vi "HEWH RLT PRAT.vi"() -> ()   [LabVIEW 2023] (continued)
            n517 = call <vilib>:"Add State(s) to Queue__jki_lib_state_machine.vi"("State(s) in (\"\")"=w1428) -> ("States Out"=w1427:string)  [unwired: 14 in]
          }
          frame "Data: Update Data Path C" {
            n518 = Unbundle By Name(w1451) -> ("Display Data (RLT).Station Label Display"=w1450:string)
            n519 = case shown="True" "New File Per CycC" {
              tunnel: w1456 -> [w1461 w1479]
              tunnel: w1455 -> [w1462 w1471]
              tunnel: [w1462 w1470] -> w1454
              tunnel: [w1460 w1467] -> w1453
              tunnel: w1450 -> [_ w1465]
              frame False {
                n520 = Bundle By Name(cluster=w1461, "File Locations C.New Summary Created"=FALSE) -> (w1460:T88)
              }
              frame True {
                # "I re-purposed this control. It now\ntriggers a header write in \"Data:\nSave\""
                # "I couldnt use a local to pass data due to UI Button"
                n521 = local read "Appliance Details C"() -> (w1464:T5)
                n522 = property on="Cycle Count Display" class="DigNum (strict)"() -> ("Value"=w1466:i32)  [unwired: 2 in, 2 out]
                n523 = Unbundle By Name(w1479) -> ("Core HEWH Data Input C.LV Program"=w1463:T25, "File Locations C"=w1474:T3)
                n524 = Unbundle By Name(w1464) -> ("Appliance Common.TR Number:"=w1477:string, "Appliance Common.Lab ID:"=w1476:string, "Appliance Common.Serial Number:"=w1475:string)
                n525 = Bundle By Name(cluster=T31 {"Appliance Details"={"FileVersionInfo"={"FileVersion"="", "ProductName"="", "InternalName"="", "CompanyName"="", "LegalCopyright"="", "FileDescription"=""}, "Dishwasher Info"={"Open Cup Weight (gm):"=0.0, "Auto Cup Weight (gm):"=0.0, "Detergent-Dish:"="", "Inlet Temperature-Dish:"="", "Cycle Mode-Dish:"="", "Unit Control-Dish:"="", "Manufacturer-Dish:"=""}, "Washer Info"={"Hot Water Temperature (Fahrenheit):"="", "Cold Water Temperature (Fahrenheit):"="", "Capacity (cu.ft):"=0.0, "Initial Cloth Weight:"=0.0, "Cloth Lot:"=0, "Model Family:"="", "Program Name:"="", "Cycle Selection:"="", "Wash Temperature:"="", "Rinse Temperature:"="", "Load Size:"=""}, "File Name Output Array"=[], "Calibration Output Array"=[], "Appliance Common"={"Engineer:"="", "Model Number:"="", "Serial Number:"="", "Comments:"="", "Station ID:"="", "Technician:"="", "TR Number:"="", "Lab ID:"="", "Voltage:"="", "Water Pressure (PSI):"="", "Test Date:"="", "Computer Name:"="", "IP Address:"="", "Ambient RH:"="", "Frequency:"="", "Build:"="", "Filename:"="", "Test Type:"="", "Load Run #:"=0, "Ambient Temperature (F):"="", "File Path:"=path "", "Cycles Per Year"=60}, "Water Heater"={"Heating Mode:"=""}, "Dryer"={"Heat Setting:"="", "Washer Water Temperature (60 ± 5°F):"=60, "Water Hardness (PPM):"=17, "Dryness Setting:"="", "Dryer Type:"="", "Exhaust:"="", "Drying Cycle:"="", "Load Type:"="", "Nominal Load Weight"="", "Dryer Initial IMC Data"={"Measured IMC (lbs)"=7.0, "Actual Initial RMC (%)"=7.0, "RMC (Desired %)"=100.0, "Bone Dry Wt(lbs)"=7.0, "Tolerance(%)"=5.0, "Actual Final RMC (%)"=0.0, "CEF (lbf/kWh)"=0.0, "Minimum Weight (lbf)"=0.0, "Average Weight (lbf)"=0.0, "Maximum Weight (lbf)"=0.0, "Measured IMC In Range?"=FALSE, "Moisture Reduction Factor"=55.5, "Field Use Factor"=1.04, "Empty Dryer Cold Weigth"=0.0, "Energy Standard"=enum."D2-Automatic Dryer", "Weight Cloth (lbs)"=0.0, "Relative Moisture Content (%)"=0.0, "Relative Moisture Content - Avg (%)"=0.0}}}, "Display Data (RLT)"={"Status Color"=0, "Serial Number Display"="", "Cycle Count Display"=0, "Station Label Display"="", "Current Run Start Time Display"=0.0, "Board ID Display"="", "RPM Display"=0, "Current Display"=0.0, "Current Path Display"=path "", "Saving Display"=FALSE, "Unit Type Display"=enum."", "Total Time On Display"=0.0, "UI Button"=FALSE}} ("Initialize.Washer In"), "Appliance Details.Appliance Common.TR Number:"=w1477, "Appliance Details.Appliance Common.Lab ID:"=w1476, "Appliance Details.Appliance Common.Serial Number:"=w1475, "Display Data (RLT).Station Label Display"=w1465, "Display Data (RLT).Cycle Count Display"=w1466) -> (w1473:T31)
                n526 = call "Save File Format All Folders.vi"("LV Program"=w1463, "error in (no error)"=w1471, "Initialize.Washer In"=w1473, "File Locations In"=w1474) -> ("error out"=w1470:errorcluster, "New File?"=w1469:bool, "File Locations Out"=w1472:T3)  [unwired: 5 in]
                n527 = Bundle By Name(cluster=w1479, "File Locations C"=w1472) -> (w1468:T88)
                n528 = Bundle By Name(cluster=w1468, "File Locations C.New Summary Created"=w1469) -> (w1467:T88)
              }
            }
            n529 = call <vilib>:"Add State(s) to Queue__jki_lib_state_machine.vi"("State(s) in (\"\")"=w1458) -> ("States Out"=w1457:string)  [unwired: 14 in]
          }
          frame "Data: Update Data Path D" {
            n530 = case shown="True" "New File Per CycD" {
              tunnel: w1485 -> [w1490 w1509]
              tunnel: w1484 -> [w1491 w1501]
              tunnel: [w1491 w1500] -> w1483
              tunnel: [w1489 w1497] -> w1482
              tunnel: w1480 -> [_ w1494]
              frame False {
                n531 = Bundle By Name(cluster=w1490, "File Locations D.New Summary Created"=FALSE) -> (w1489:T88)
              }
              frame True {
                # "I re-purposed this control. It now\ntriggers a header write in \"Data:\nSave\""
                # "I couldnt use a local to pass data due to UI Button"
                n532 = local read "Appliance Details D"() -> (w1495:T5)
                n533 = Unbundle By Name(w1494) -> ("Display Data (RLT).Station Label Display"=w1493:string)
                n534 = property on="Cycle Count Display" class="DigNum (strict)"() -> ("Value"=w1496:i32)  [unwired: 2 in, 2 out]
                n535 = Unbundle By Name(w1509) -> ("Core HEWH Data Input D.LV Program"=w1492:T25, "File Locations D"=w1504:T3)
                n536 = Unbundle By Name(w1495) -> ("Appliance Common.TR Number:"=w1507:string, "Appliance Common.Lab ID:"=w1506:string, "Appliance Common.Serial Number:"=w1505:string)
                n537 = Bundle By Name(cluster=T31 {"Appliance Details"={"FileVersionInfo"={"FileVersion"="", "ProductName"="", "InternalName"="", "CompanyName"="", "LegalCopyright"="", "FileDescription"=""}, "Dishwasher Info"={"Open Cup Weight (gm):"=0.0, "Auto Cup Weight (gm):"=0.0, "Detergent-Dish:"="", "Inlet Temperature-Dish:"="", "Cycle Mode-Dish:"="", "Unit Control-Dish:"="", "Manufacturer-Dish:"=""}, "Washer Info"={"Hot Water Temperature (Fahrenheit):"="", "Cold Water Temperature (Fahrenheit):"="", "Capacity (cu.ft):"=0.0, "Initial Cloth Weight:"=0.0, "Cloth Lot:"=0, "Model Family:"="", "Program Name:"="", "Cycle Selection:"="", "Wash Temperature:"="", "Rinse Temperature:"="", "Load Size:"=""}, "File Name Output Array"=[], "Calibration Output Array"=[], "Appliance Common"={"Engineer:"="", "Model Number:"="", "Serial Number:"="", "Comments:"="", "Station ID:"="", "Technician:"="", "TR Number:"="", "Lab ID:"="", "Voltage:"="", "Water Pressure (PSI):"="", "Test Date:"="", "Computer Name:"="", "IP Address:"="", "Ambient RH:"="", "Frequency:"="", "Build:"="", "Filename:"="", "Test Type:"="", "Load Run #:"=0, "Ambient Temperature (F):"="", "File Path:"=path "", "Cycles Per Year"=60}, "Water Heater"={"Heating Mode:"=""}, "Dryer"={"Heat Setting:"="", "Washer Water Temperature (60 ± 5°F):"=60, "Water Hardness (PPM):"=17, "Dryness Setting:"="", "Dryer Type:"="", "Exhaust:"="", "Drying Cycle:"="", "Load Type:"="", "Nominal Load Weight"="", "Dryer Initial IMC Data"={"Measured IMC (lbs)"=7.0, "Actual Initial RMC (%)"=7.0, "RMC (Desired %)"=100.0, "Bone Dry Wt(lbs)"=7.0, "Tolerance(%)"=5.0, "Actual Final RMC (%)"=0.0, "CEF (lbf/kWh)"=0.0, "Minimum Weight (lbf)"=0.0, "Average Weight (lbf)"=0.0, "Maximum Weight (lbf)"=0.0, "Measured IMC In Range?"=FALSE, "Moisture Reduction Factor"=55.5, "Field Use Factor"=1.04, "Empty Dryer Cold Weigth"=0.0, "Energy Standard"=enum."D2-Automatic Dryer", "Weight Cloth (lbs)"=0.0, "Relative Moisture Content (%)"=0.0, "Relative Moisture Content - Avg (%)"=0.0}}}, "Display Data (RLT)"={"Status Color"=0, "Serial Number Display"="", "Cycle Count Display"=0, "Station Label Display"="", "Current Run Start Time Display"=0.0, "Board ID Display"="", "RPM Display"=0, "Current Display"=0.0, "Current Path Display"=path "", "Saving Display"=FALSE, "Unit Type Display"=enum."", "Total Time On Display"=0.0, "UI Button"=FALSE}} ("Initialize.Washer In"), "Appliance Details.Appliance Common.TR Number:"=w1507, "Appliance Details.Appliance Common.Lab ID:"=w1506, "Appliance Details.Appliance Common.Serial Number:"=w1505, "Display Data (RLT).Station Label Display"=w1493, "Display Data (RLT).Cycle Count Display"=w1496) -> (w1503:T31)
                n538 = call "Save File Format All Folders.vi"("LV Program"=w1492, "error in (no error)"=w1501, "Initialize.Washer In"=w1503, "File Locations In"=w1504) -> ("error out"=w1500:errorcluster, "New File?"=w1499:bool, "File Locations Out"=w1502:T3)  [unwired: 5 in]
                n539 = Bundle By Name(cluster=w1509, "File Locations D"=w1502) -> (w1498:T88)
                n540 = Bundle By Name(cluster=w1498, "File Locations D.New Summary Created"=w1499) -> (w1497:T88)
              }
            }
            n541 = call <vilib>:"Add State(s) to Queue__jki_lib_state_machine.vi"("State(s) in (\"\")"=w1487) -> ("States Out"=w1486:string)  [unwired: 14 in]
          }
          frame "Data: Update RLT Channels" {
            # "Update the RLT Station Channels Control"
            n542 = Unbundle By Name(w1538) -> ("Core HEWH Data Input A.LV Program"=w1534:T25, "A Data Array"=w1518:string[][], "B Data Array"=w1517:string[][], "C Data Array"=w1516:string[][], "D Data Array"=w1515:string[][], "File Locations A"=w1537:T3, "File Locations B"=w1536:T3, "File Locations C"=w1510:T3, "File Locations D"=w1535:T3, "Core HEWH Data Input D"=w1523:T13, "Core HEWH Data Input C"=w1525:T13, "Core HEWH Data Input B"=w1526:T13, "Core HEWH Data Input A"=w1527:T13)
            "Station A" <- w1518
            "Station B" <- w1517
            "Station C" <- w1516
            "Station D" <- w1515
            "Station A SO Display" <- w1518
            "Station B SO Display" <- w1517
            "Station C SO Display" <- w1516
            "Station D SO Display" <- w1515
            n543 = local read "Condition B"() -> (w1513:T2)
            n544 = local read "Condition A"() -> (w1514:T2)
            n545 = local read "Station D Test Sequence"() -> (w1519:T15[])
            n546 = local read "Station A Test Sequence"() -> (w1522:T15[])
            n547 = local read "Station B Test Sequence"() -> (w1521:T15[])
            n548 = local read "Current Draw Parameters"() -> (w1532:T48)
            n549 = local read "Station C Test Sequence"() -> (w1520:T15[])
            n550 = call <vilib>:"Add State(s) to Queue__jki_lib_state_machine.vi"("State(s) in (\"\")"=w1540) -> ("States Out"=w1539:string)  [unwired: 14 in]
            n551 = local read "Condition C"() -> (w1512:T2)
            n552 = local read "Condition D"() -> (w1511:T2)
            n553 = local write "File Locations A"(w1537) -> ()
            n554 = local write "File Locations B"(w1536) -> ()
            n555 = local write "File Locations C"(w1510) -> ()
            n556 = local write "File Locations D"(w1535) -> ()
            n557 = call "HEWH Update Draw Sequence Data.vi"("Core HEWH Data Input A"=w1527, "Station A Test Sequence"=w1522, "Condition B"=w1513, "Station B Test Sequence"=w1521, "Draw Parameters"=w1532, "error in (no error)"=w1533, "Core HEWH Data Input B"=w1526, "Station C Test Sequence"=w1520, "Condition A"=w1514, "Condition C"=w1512, "Core HEWH Data Input C"=w1525, "Station D Test Sequence"=w1519, "Core HEWH Data Input D"=w1523, "Condition D"=w1511) -> ("Core HEWH Data Output"=w1528:T13, "Core HEWH Data Output 2"=w1529:T13, "Core HEWH Data Output 3"=w1530:T13, "Core HEWH Data Output 4"=w1531:T13, "error out"=w1524:errorcluster)  [unwired: 1 in]
            n558 = case shown="\"HEWH RLT\"" w1534 {
              tunnel: w1518 -> [_ w1552]
              tunnel: w1517 -> [_ w1549]
              tunnel: w1516 -> [_ w1548]
              tunnel: w1515 -> [_ w1547]
              frame Default {
              }
              frame "HEWH RLT" {
                n559 = local read "DAQ for B"() -> (w1546:bool)
                n560 = local read "DAQ for D"() -> (w1544:bool)
                n561 = local read "DAQ for A"() -> (w1551:bool)
                n562 = local read "DAQ for C"() -> (w1545:bool)
                n563 = call "HEWH RLT Get Current.vi"("DAQ for A"=w1551, "A Data Array"=w1552) -> ("Current"=w1550:dbl)  [unwired: 8 in, 1 out]
                n564 = call "HEWH RLT Get Current.vi"("DAQ for A"=w1546, "A Data Array"=w1549) -> ("Current"=w1543:dbl)  [unwired: 8 in, 1 out]
                n565 = call "HEWH RLT Get Current.vi"("DAQ for A"=w1545, "A Data Array"=w1548) -> ("Current"=w1542:dbl)  [unwired: 8 in, 1 out]
                n566 = call "HEWH RLT Get Current.vi"("DAQ for A"=w1544, "A Data Array"=w1547) -> ("Current"=w1541:dbl)  [unwired: 8 in, 1 out]
                n567 = local write "Current (D)"(w1541) -> ()
                n568 = local write "Current (A)"(w1550) -> ()
                n569 = local write "Current (B)"(w1543) -> ()
                n570 = local write "Current (C)"(w1542) -> ()
              }
            }
            n571 = local write "Core HEWH Data Input B"(w1529) -> ()
            n572 = local write "Core HEWH Data Input A"(w1528) -> ()
            n573 = local write "Core HEWH Data Input C"(w1530) -> ()
            n574 = local write "Core HEWH Data Input D"(w1531) -> ()
          }
          frame "Show Data A" {
            n575 = Unbundle By Name(w1568) -> ("Plot Array A"=w1571:dbl[][], "A Data Array"=w1561:string[][], "File Locations A.New Summary Created"=w1562:bool, "Core HEWH Data Input A.LV Program"=w1554:T25)
            n576 = call <vilib>:"Add State(s) to Queue__jki_lib_state_machine.vi"("State(s) in (\"\")"=w1573) -> ("States Out"=w1572:string)  [unwired: 14 in]
            n577 = Transpose 2D Array(2D array=w1561) -> (transposed array=w1560:string[][])
            n578 = case shown="Default" w1554 {
              tunnel: [TRUE ("Reset After 24hrs") FALSE ("Reset After 24hrs")] -> w1555
              frame Default {
              }
              frame "PRAT", "HEWH RLT" {
              }
            }
            n579 = call "UTILITY Create Plot Array.vi"("Save Data"=w1560, "Plot Array in"=w1571) -> ("Plot Array out"=w1559:dbl[][])  [unwired: 8 in, 1 out]
            n580 = call "UTILITY MultiPlot.vi"("Y-Axis-2"="Y-Axis2 - Station A", "Y-Axis-1"="Y-Axis1 - Station A", "X-Axis"="X-Axis - Station A", "Save Data"=w1560, "Plot Array"=w1571) -> ("Plot Cluster"=w1569:T37)  [unwired: 5 in, 1 out]
            n581 = case shown="False" "Pause Graph" {
              tunnel: w1569 -> [w1580 _]
              tunnel: "X-Axis - Station A" -> [w1579 _]
              tunnel: "Y-Axis1 - Station A" -> [w1578 _]
              frame False {
                n582 = property on="XY Graph - Station A" class="XYGraph (strict)"("XScale.NameLbl.Text"=w1579, "YScale.NameLbl.Text"=w1578) -> ()  [unwired: 2 in, 2 out]
                "XY Graph - Station A" <- w1580
              }
              frame True {
              }
            }
            n583 = call "UTILITY Array Reset.vi"("Reset After 24hrs"=w1555, "Plot Array Input"=w1559) -> ("Reset Array"=w1558:bool)  [unwired: 9 in]
            n584 = Compound Arithmetic op=OR("Clear Graph Data", w1562, w1558) -> (w1563:bool)
            n585 = case shown="False" w1563 {
              tunnel: w1559 -> [w1576 _]
              tunnel: [w1576 dbl[][] [] ("Plot Array out")] -> w1566
              frame False {
              }
              frame True {
              }
            }
            n586 = Bundle By Name(cluster=w1568, "Plot Array A"=w1566) -> (w1567:T88)
          }
          frame "Show Data B" {
            n587 = Unbundle By Name(w1593) -> ("Plot Array B"=w1591:dbl[][], "B Data Array"=w1588:string[][], "File Locations B.New Summary Created"=w1590:bool, "Core HEWH Data Input B.LV Program"=w1582:T25)
            n588 = Transpose 2D Array(2D array=w1588) -> (transposed array=w1587:string[][])
            n589 = call <vilib>:"Add State(s) to Queue__jki_lib_state_machine.vi"("State(s) in (\"\")"=w1601) -> ("States Out"=w1600:string)  [unwired: 14 in]
            n590 = case shown="Default" w1582 {
              tunnel: [TRUE ("Reset After 24hrs") FALSE ("Reset After 24hrs")] -> w1581
              frame Default {
              }
              frame "PRAT", "HEWH RLT" {
              }
            }
            n591 = call "UTILITY Create Plot Array.vi"("Save Data"=w1587, "Plot Array in"=w1591) -> ("Plot Array out"=w1586:dbl[][])  [unwired: 8 in, 1 out]
            n592 = call "UTILITY MultiPlot.vi"("Y-Axis-2"="Y-Axis2 - Station B", "Y-Axis-1"="Y-Axis1 - Station B", "X-Axis"="X-Axis - Station B", "Save Data"=w1587, "Plot Array"=w1591) -> ("Plot Cluster"=w1598:T37)  [unwired: 5 in, 1 out]
            n593 = case shown="False" "Pause Graph B" {
              tunnel: w1598 -> [w1608 _]
              tunnel: "X-Axis - Station B" -> [w1607 _]
              tunnel: "Y-Axis1 - Station B" -> [w1606 _]
              frame False {
                n594 = property on="XY Graph - Station B" class="XYGraph (strict)"("XScale.NameLbl.Text"=w1607, "YScale.NameLbl.Text"=w1606) -> ()  [unwired: 2 in, 2 out]
                "XY Graph - Station B" <- w1608
              }
              frame True {
              }
            }
            n595 = call "UTILITY Array Reset.vi"("Reset After 24hrs"=w1581, "Plot Array Input"=w1586) -> ("Reset Array"=w1585:bool)  [unwired: 9 in]
            n596 = Compound Arithmetic op=OR("Clear Graph Data B", w1590, w1585) -> (w1594:bool)
            n597 = case shown="False" w1594 {
              tunnel: w1586 -> [w1604 _]
              tunnel: [w1604 dbl[][] [] ("Plot Array out")] -> w1597
              frame False {
              }
              frame True {
              }
            }
            n598 = Bundle By Name(cluster=w1593, "Plot Array B"=w1597) -> (w1592:T88)
          }
          frame "Show Data C" {
            n599 = Unbundle By Name(w1619) -> ("Plot Array C"=w1621:dbl[][], "C Data Array"=w1616:string[][], "File Locations C.New Summary Created"=w1617:bool, "Core HEWH Data Input C.LV Program"=w1610:T25)
            n600 = Transpose 2D Array(2D array=w1616) -> (transposed array=w1615:string[][])
            n601 = call <vilib>:"Add State(s) to Queue__jki_lib_state_machine.vi"("State(s) in (\"\")"=w1629) -> ("States Out"=w1628:string)  [unwired: 14 in]
            n602 = case shown="Default" w1610 {
              tunnel: [TRUE ("Reset After 24hrs") FALSE ("Reset After 24hrs")] -> w1609
              frame Default {
              }
              frame "PRAT", "HEWH RLT" {
              }
            }
            n603 = call "UTILITY Create Plot Array.vi"("Save Data"=w1615, "Plot Array in"=w1621) -> ("Plot Array out"=w1614:dbl[][])  [unwired: 8 in, 1 out]
            n604 = call "UTILITY MultiPlot.vi"("Y-Axis-2"="Y-Axis2 - Station C", "Y-Axis-1"="Y-Axis1 - Station C", "X-Axis"="X-Axis - Station C", "Save Data"=w1615, "Plot Array"=w1621) -> ("Plot Cluster"=w1626:T37)  [unwired: 5 in, 1 out]
            n605 = call "UTILITY Array Reset.vi"("Reset After 24hrs"=w1609, "Plot Array Input"=w1614) -> ("Reset Array"=w1613:bool)  [unwired: 9 in]
            n606 = case shown="False" "Pause Graph C" {
              tunnel: w1626 -> [w1636 _]
              tunnel: "X-Axis - Station C" -> [w1635 _]
              tunnel: "Y-Axis1 - Station C" -> [w1634 _]
              frame False {
                n607 = property on="XY Graph - Station C" class="XYGraph (strict)"("XScale.NameLbl.Text"=w1635, "YScale.NameLbl.Text"=w1634) -> ()  [unwired: 2 in, 2 out]
                "XY Graph - Station C" <- w1636
              }
              frame True {
              }
            }
            n608 = Compound Arithmetic op=OR("Clear Graph Data C", w1617, w1613) -> (w1622:bool)
            n609 = case shown="False" w1622 {
              tunnel: w1614 -> [w1632 _]
              tunnel: [w1632 dbl[][] [] ("Plot Array out")] -> w1625
              frame False {
              }
              frame True {
              }
            }
            n610 = Bundle By Name(cluster=w1619, "Plot Array C"=w1625) -> (w1618:T88)
          }
          frame "Show Data D" {
            n611 = Unbundle By Name(w1649) -> ("Plot Array D"=w1647:dbl[][], "D Data Array"=w1645:string[][], "File Locations D.New Summary Created"=w1646:bool, "Core HEWH Data Input D.LV Program"=w1638:T25)
            n612 = call <vilib>:"Add State(s) to Queue__jki_lib_state_machine.vi"("State(s) in (\"\")"=w1657) -> ("States Out"=w1656:string)  [unwired: 14 in]
            n613 = case shown="Default" w1638 {
              tunnel: [TRUE ("Reset After 24hrs") FALSE ("Reset After 24hrs")] -> w1637
              frame Default {
              }
              frame "PRAT", "HEWH RLT" {
              }
            }
            n614 = Transpose 2D Array(2D array=w1645) -> (transposed array=w1644:string[][])
            n615 = call "UTILITY Create Plot Array.vi"("Save Data"=w1644, "Plot Array in"=w1647) -> ("Plot Array out"=w1643:dbl[][])  [unwired: 8 in, 1 out]
            n616 = call "UTILITY MultiPlot.vi"("Y-Axis-2"="Y-Axis2 - Station D", "Y-Axis-1"="Y-Axis1 - Station D", "X-Axis"="X-Axis - Station D", "Save Data"=w1644, "Plot Array"=w1647) -> ("Plot Cluster"=w1654:T37)  [unwired: 5 in, 1 out]
            n617 = call "UTILITY Array Reset.vi"("Reset After 24hrs"=w1637, "Plot Array Input"=w1643) -> ("Reset Array"=w1642:bool)  [unwired: 9 in]
            n618 = case shown="False" "Pause Graph D" {
              tunnel: w1654 -> [w1664 _]
              tunnel: "X-Axis - Station D" -> [w1663 _]
              tunnel: "Y-Axis1 - Station D" -> [w1662 _]
              frame False {
                n619 = property on="XY Graph - Station D" class="XYGraph (strict)"("XScale.NameLbl.Text"=w1663, "YScale.NameLbl.Text"=w1662) -> ()  [unwired: 2 in, 2 out]
                "XY Graph - Station D" <- w1664
              }
              frame True {
              }
            }
            n620 = Compound Arithmetic op=OR("Clear Graph Data D", w1646, w1642) -> (w1650:bool)
            n621 = case shown="False" w1650 {
              tunnel: w1643 -> [w1660 _]
              tunnel: [w1660 dbl[][] [] ("Plot Array out")] -> w1653
              frame False {
              }
              frame True {
              }
            }
            n622 = Bundle By Name(cluster=w1649, "Plot Array D"=w1653) -> (w1648:T88)
          }
          frame "Data: Save Data" {
            # "Probably better to pull the whole control in. Would just have to do some event sequencing...guess this is lazy"
            n623 = local read "Appliance Details B"() -> (w1668:T5)
            n624 = local read "Appliance Details D"() -> (w1666:T5)
            n625 = local read "Log Data Output (D)"() -> (w1670:bool)
            n626 = Unbundle By Name(w1690) -> ("File Locations A"=w1685:T3, "File Locations B"=w1684:T3, "File Locations C"=w1683:T3, "File Locations D"=w1682:T3, "A Data Array"=w1681:string[][], "B Data Array"=w1680:string[][], "C Data Array"=w1679:string[][], "D Data Array"=w1678:string[][])
            n627 = local read "Appliance Details A"() -> (w1669:T5)
            n628 = local read "Appliance Details C"() -> (w1667:T5)
            n629 = local read "Log Data Output (C)"() -> (w1671:bool)
            n630 = local read "Log Data Output (B)"() -> (w1672:bool)
            n631 = local read "Log Data Output (A)"() -> (w1673:bool)
            n632 = Build Array(w1669, w1668, w1667, w1666) -> (w1665:T5[])
            n633 = call "Save File Four Stations.vi"("File Locations A in"=w1685, "File Locations B in"=w1684, "File Locations C in"=w1683, "File Locations D in"=w1682, "Save Data A"=w1673, "A Data Array"=w1681, "Save Data B"=w1672, "B Data Array"=w1680, "Save Data C"=w1671, "C Data Array"=w1679, "Save Data D"=w1670, "D Data Array"=w1678, "Appliance Details"=w1665) -> ("Saving A"=w1677:bool, "File Locations A out"=w1689:T3, "File Locations B out"=w1688:T3, "File Locations C out"=w1687:T3, "File Locations D out"=w1686:T3, "Saving B"=w1676:bool, "Saving C"=w1675:bool, "Saving D"=w1674:bool)  [unwired: 6 in, 1 out]
            n634 = Bundle By Name(cluster=w1690, "File Locations A"=w1689, "File Locations B"=w1688, "File Locations C"=w1687, "File Locations D"=w1686) -> (w1691:T88)
            n635 = property on="Saving Display" class="Bool (strict)"("Value"=w1677) -> ()  [unwired: 2 in, 2 out]
            n636 = property on="Saving Display" class="Bool (strict)"("Value"=w1676) -> ()  [unwired: 2 in, 2 out]
            n637 = property on="Saving Display" class="Bool (strict)"("Value"=w1675) -> ()  [unwired: 2 in, 2 out]
            n638 = property on="Saving Display" class="Bool (strict)"("Value"=w1674) -> ()  [unwired: 2 in, 2 out]
            n639 = call <vilib>:"Add State(s) to Queue__jki_lib_state_machine.vi"("State(s) in (\"\")"=w1694) -> ("States Out"=w1693:string)  [unwired: 14 in]
          }
          frame "Add Final Data A" {
            n640 = Unbundle By Name(w1703) -> ("File Locations A.Data File Paths.Data File Path"=w1707:path, "Core HEWH Data Input A.Calc and Calibration.All Draw Stats"=w1706:string[][])
            "All Draw Stats" <- w1706
            n641 = call "UTILITY String Notifier.vi"("Status"=UTILITY_Notifier."Set", "error in (no error)"=w1696, "Set Status"="Writing Final Headers...", "name (unnamed)"="MessageA") -> ("error out"=w1695:errorcluster)  [unwired: 6 in, 1 out]
            n642 = call "Save File Add Summary Data.vi"("Data That Has Been\nCollecting"=w1707, "Error In"=w1695, "Use 2D String Summary"=TRUE, "Add Final RMC"=FALSE, "2D String Summary"=w1706) -> ("Error Out"=w1701:errorcluster)  [unwired: 14 in]
            n643 = flat-sequence {
              tunnel: w1703 -> [w1718]
              tunnel: [w1717] -> w1702
              tunnel: w1701 -> [w1714]
              tunnel: [w1713] -> w1700
              frame #0 {
                w1710 = FALSE ("Value")
                # "Used in auto test portion.\nTired of tinkering with\nevents"
                n644 = property on="Saving Display" class="Bool (strict)"("Value"=w1710) -> ()  [unwired: 2 in, 2 out]
                n645 = local write "Final Headers A"(w1710) -> ()
                n646 = Bundle By Name(cluster=w1718, "File Locations A.Data File Paths"=T4 {"Data File Path"=path "", "Debug File Path"=path "", "Bus Log Path"=path "", "Current"=path "", "Summary"=path ""} ("Data File Paths")) -> (w1717:T88)
                n647 = call "UTILITY String Notifier.vi"("Status"=UTILITY_Notifier."Set", "error in (no error)"=w1714, "Set Status"="", "name (unnamed)"="MessageA") -> ("error out"=w1713:errorcluster)  [unwired: 6 in, 1 out]
              }
            }
            n648 = call <vilib>:"Add State(s) to Queue__jki_lib_state_machine.vi"("State(s) in (\"\")"=w1709) -> ("States Out"=w1708:string)  [unwired: 14 in]
          }
          frame "Add Final Data B" {
            n649 = Unbundle By Name(w1726) -> ("File Locations B.Data File Paths.Data File Path"=w1731:path, "Core HEWH Data Input B.Calc and Calibration.All Draw Stats"=w1730:string[][])
            n650 = call "UTILITY String Notifier.vi"("Status"=UTILITY_Notifier."Set", "error in (no error)"=w1720, "Set Status"="Writing Final Headers...", "name (unnamed)"="MessageB") -> ("error out"=w1719:errorcluster)  [unwired: 6 in, 1 out]
            n651 = call "Save File Add Summary Data.vi"("Data That Has Been\nCollecting"=w1731, "Error In"=w1719, "Use 2D String Summary"=TRUE, "Add Final RMC"=FALSE, "2D String Summary"=w1730) -> ("Error Out"=w1727:errorcluster)  [unwired: 14 in]
            n652 = flat-sequence {
              tunnel: w1726 -> [w1742]
              tunnel: [w1741] -> w1725
              tunnel: w1727 -> [w1738]
              tunnel: [w1737] -> w1724
              frame #0 {
                w1734 = FALSE ("Value")
                n653 = property on="Saving Display" class="Bool (strict)"("Value"=w1734) -> ()  [unwired: 2 in, 2 out]
                n654 = local write "Final Headers B"(w1734) -> ()
                n655 = Bundle By Name(cluster=w1742, "File Locations B.Data File Paths"=T4 {"Data File Path"=path "", "Debug File Path"=path "", "Bus Log Path"=path "", "Current"=path "", "Summary"=path ""} ("Data File Paths")) -> (w1741:T88)
                n656 = call "UTILITY String Notifier.vi"("Status"=UTILITY_Notifier."Set", "error in (no error)"=w1738, "Set Status"="", "name (unnamed)"="MessageB") -> ("error out"=w1737:errorcluster)  [unwired: 6 in, 1 out]
              }
            }
            n657 = call <vilib>:"Add State(s) to Queue__jki_lib_state_machine.vi"("State(s) in (\"\")"=w1733) -> ("States Out"=w1732:string)  [unwired: 14 in]
          }
          frame "Add Final Data C" {
            n658 = Unbundle By Name(w1750) -> ("File Locations C.Data File Paths.Data File Path"=w1755:path, "Core HEWH Data Input C.Calc and Calibration.All Draw Stats"=w1754:string[][])
            n659 = call "UTILITY String Notifier.vi"("Status"=UTILITY_Notifier."Set", "error in (no error)"=w1744, "Set Status"="Writing Final Headers...", "name (unnamed)"="MessageC") -> ("error out"=w1743:errorcluster)  [unwired: 6 in, 1 out]
            n660 = call "Save File Add Summary Data.vi"("Data That Has Been\nCollecting"=w1755, "Error In"=w1743, "Use 2D String Summary"=TRUE, "Add Final RMC"=FALSE, "2D String Summary"=w1754) -> ("Error Out"=w1751:errorcluster)  [unwired: 14 in]
            n661 = flat-sequence {
              tunnel: w1750 -> [w1766]
              tunnel: [w1765] -> w1749
              tunnel: w1751 -> [w1762]
              tunnel: [w1761] -> w1748
              frame #0 {
                w1758 = FALSE ("Value")
                n662 = local write "Final Headers C"(w1758) -> ()
                n663 = Bundle By Name(cluster=w1766, "File Locations C.Data File Paths"=T4 {"Data File Path"=path "", "Debug File Path"=path "", "Bus Log Path"=path "", "Current"=path "", "Summary"=path ""} ("Data File Paths")) -> (w1765:T88)
                n664 = property on="Saving Display" class="Bool (strict)"("Value"=w1758) -> ()  [unwired: 2 in, 2 out]
                n665 = call "UTILITY String Notifier.vi"("Status"=UTILITY_Notifier."Set", "error in (no error)"=w1762, "Set Status"="", "name (unnamed)"="MessageC") -> ("error out"=w1761:errorcluster)  [unwired: 6 in, 1 out]
              }
            }
            n666 = call <vilib>:"Add State(s) to Queue__jki_lib_state_machine.vi"("State(s) in (\"\")"=w1757) -> ("States Out"=w1756:string)  [unwired: 14 in]
          }
          frame "Add Final Data D" {
            n667 = Unbundle By Name(w1774) -> ("File Locations D.Data File Paths.Data File Path"=w1779:path, "Core HEWH Data Input D.Calc and Calibration.All Draw Stats"=w1778:string[][])
            n668 = call "UTILITY String Notifier.vi"("Status"=UTILITY_Notifier."Set", "error in (no error)"=w1769, "Set Status"="Writing Final Headers...", "name (unnamed)"="MessageD") -> ("error out"=w1768:errorcluster)  [unwired: 6 in, 1 out]
            n669 = call "Save File Add Summary Data.vi"("Data That Has Been\nCollecting"=w1779, "Error In"=w1768, "Use 2D String Summary"=TRUE, "Add Final RMC"=FALSE, "2D String Summary"=w1778) -> ("Error Out"=w1775:errorcluster)  [unwired: 14 in]
            n670 = flat-sequence {
              tunnel: w1774 -> [w1790]
              tunnel: [w1789] -> w1773
              tunnel: w1775 -> [w1786]
              tunnel: [w1785] -> w1772
              frame #0 {
                w1782 = FALSE ("Value")
                n671 = property on="Saving Display" class="Bool (strict)"("Value"=w1782) -> ()  [unwired: 2 in, 2 out]
                n672 = local write "Final Headers D"(w1782) -> ()
                n673 = Bundle By Name(cluster=w1790, "File Locations D.Data File Paths"=T4 {"Data File Path"=path "", "Debug File Path"=path "", "Bus Log Path"=path "", "Current"=path "", "Summary"=path ""} ("Data File Paths")) -> (w1789:T88)
                n674 = call "UTILITY String Notifier.vi"("Status"=UTILITY_Notifier."Set", "error in (no error)"=w1786, "Set Status"="", "name (unnamed)"="MessageD") -> ("error out"=w1785:errorcluster)  [unwired: 6 in, 1 out]
              }
            }
            n675 = call <vilib>:"Add State(s) to Queue__jki_lib_state_machine.vi"("State(s) in (\"\")"=w1781) -> ("States Out"=w1780:string)  [unwired: 14 in]
          }
          frame "-----Simple Processing-----" {
          }
          frame "Calculate Max AVG TC Temp" {
            n676 = Unbundle By Name(w1799) -> ("Core HEWH Data Input A"=w1818:T13, "Core HEWH Data Input B"=w1813:T13, "Core HEWH Data Input C"=w1807:T13, "Core HEWH Data Input D"=w1803:T13)
            n677 = local read "Current Draw Parameters"() -> (w1802:T48)
            n678 = call "HEWH Temp Decline Main.vi"("Station ID"="A", "error in (no error)"=w1817, "Temperature Decline Amount (°F)"="Temperature Decline Amount (°F)", "Core HEWH Data Input A"=w1818, "Current Draw Parameters"=w1802) -> ("error out"=w1815:errorcluster, "Core HEWH Data Output"=w1797:T13, "Temp Decline Complete"=→"Temp Decline Complete A":bool)  [unwired: 4 in]
            n679 = call "HEWH Temp Decline Main.vi"("Station ID"="B", "error in (no error)"=w1815, "Temperature Decline Amount (°F)"="Temperature Decline Amount (°F)", "Core HEWH Data Input A"=w1813, "Current Draw Parameters"=w1802) -> ("error out"=w1810:errorcluster, "Core HEWH Data Output"=w1796:T13, "Temp Decline Complete"=→"Temp Decline Complete B":bool)  [unwired: 4 in]
            n680 = call "HEWH Temp Decline Main.vi"("Station ID"="C", "error in (no error)"=w1810, "Temperature Decline Amount (°F)"="Temperature Decline Amount (°F)", "Core HEWH Data Input A"=w1807, "Current Draw Parameters"=w1802) -> ("error out"=w1806:errorcluster, "Core HEWH Data Output"=w1795:T13, "Temp Decline Complete"=→"Temp Decline Complete C":bool)  [unwired: 4 in]
            n681 = call "HEWH Temp Decline Main.vi"("Station ID"="D", "error in (no error)"=w1806, "Temperature Decline Amount (°F)"="Temperature Decline Amount (°F)", "Core HEWH Data Input A"=w1803, "Current Draw Parameters"=w1802) -> ("error out"=w1805:errorcluster, "Core HEWH Data Output"=w1794:T13, "Temp Decline Complete"=→"Temp Decline Complete D":bool)  [unwired: 4 in]
            n682 = Bundle By Name(cluster=w1799, "Core HEWH Data Input A"=w1797, "Core HEWH Data Input B"=w1796, "Core HEWH Data Input C"=w1795, "Core HEWH Data Input D"=w1794) -> (w1798:T88)
          }
        }
        n683 = local read "Debug"() -> (w545:bool)
        n684 = case shown="True" w545 {
          tunnel: [w559 w562] -> w544
          tunnel: w547 -> [w559 w561]
          tunnel: w546 -> [_ w560]
          frame False {
          }
          frame True {
            n685 = Build Array (concatenate)(w561, w560) -> (w562:string[])
          }
        }
        "DAQ" <- w544
        "Data Acquisition Steps Loop Count" <- w532
      }
      n686 = Unregister For Events(event registration refnum=w529, error in=w515) -> ()  [unwired: 1 out]
    }
    frame Enabled {
    }
  }
  n687 = disable-structure shown="Disabled" {
    disable-tunnel: w103 -> [w1834 _]
    disable-tunnel: w100 -> [w1831 _]
    disable-tunnel: w97 -> [w1829 _]
    disable-tunnel: w93 -> [w1828 _]
    disable-tunnel: w92 -> [w1827 _]
    disable-tunnel: w91 -> [w1826 _]
    disable-tunnel: w90 -> [w1825 _]
    disable-tunnel: w80 -> [w1824 _]
    disable-tunnel: w79 -> [w1823 _]
    disable-tunnel: w78 -> [w1822 _]
    disable-tunnel: w77 -> [w1821 _]
    disable-tunnel: w57 -> [w1820 _]
    frame Disabled {
      # "Main control algorithm"
      n688 = call <vilib>:"Add State(s) to Queue__jki_lib_state_machine.vi"("State(s) in (\"\")"=w1834) -> ("States Out"=w1837:string)  [unwired: 14 in]
      n689 = while "Main Test Process Loop" {
        shift-right: [w1859] -> _
        shift-left: _ -> [w1858]
        shift-right: [w1861] -> w1832
        shift-left: w1820 -> [w1856]
        shift-right: [w1860] -> _
        shift-left: w1837 -> [w1862]
        tunnel: [w1855] -> w1835
        shift-right: [w1854] -> _
        shift-left: string[] [] -> [w1853]
        tunnel: w1831 -> [w1850]
        tunnel: [w1849] -> w1833
        tunnel: w1829 -> [w1847]
        tunnel: w1824 -> [w1845]
        tunnel: w1823 -> [w1844]
        tunnel: w1822 -> [w1843]
        tunnel: w1821 -> [w1842]
        tunnel: w1828 -> [w1841]
        tunnel: w1827 -> [w1840]
        tunnel: w1826 -> [w1839]
        tunnel: w1825 -> [w1838]
        i -> [w1846]
        stop <- w1855 stop-if-true
        # "Main Test Process Loop"
        n690 = call <vilib>:"Parse State Queue__JKI_lib_State_Machine.vi"("State Queue"=w1862, "Error In (no error)"=w1856) -> ("Remaining States"=w1863:string, "Current State"=w1851:string, "Arguments"=w1852:string)  [unwired: 11 in]
        "Main State" <- w1851
        n691 = case shown="\"Test: Wait for Power Off (Station A)\"" w1851 {
          selector: w1851 -> [_ _ w2081 _ _ _ _ _ _ _ _ _ _ _ _ _ _ _ _ _ _ _ _ _ _ _ _ _ _ _ _ _ _ _ _ _ _ _ _]
          tunnel: w1863 -> [w1876 w2079 w2085 w2104 w2111 w2151 w2182 w2203 w2207 w2216 w2221 w2226 w2248 w2253 w2261 w2339 w2351 w2382 w2388 w2399 w2404 w2438 w2458 w2472 w2486 w2500 w2543 w2608 w2673 w2738 w2766 w2772 w2785 w2795 w2805 w2815 w2829 w2861 w2900]
          tunnel: w1852 -> [_ _ _ _ _ _ _ _ _ _ _ _ _ _ _ w2334 w2345 _ _ _ _ _ _ _ _ _ _ _ _ _ _ _ _ _ _ _ w2824 _ _]
          tunnel: w1858 -> [w1874 w2076 w2083 w2095 w2109 w2148 w2168 w2201 w2208 w2213 w2218 _ w2246 w2250 w2259 w2337 w2347 w2379 w2385 w2396 w2401 w2434 w2455 w2469 w2483 w2497 w2540 w2605 w2670 w2735 w2761 w2774 w2782 w2792 w2802 w2812 w2817 w2859 w2892]
          tunnel: [w1873 w2077 w2087 w2101 w2107 w2146 w2173 w2183 errorcluster {"status"=FALSE, "code"=0, "source"=""} ("error out") w2212 w2219 w2224 w2242 w2251 w2258 w2335 w2348 w2380 w2386 w2397 w2402 w2405 w2452 w2466 w2480 w2494 w2518 w2582 w2647 w2712 w2767 w2773 w2776 w2786 w2796 w2806 w2826 w2858 w2896] -> w1861
          tunnel: w1856 -> [w1872 w2077 w2086 w2101 w2108 w2146 w2170 w2184 w2205 w2212 w2219 w2224 w2244 w2251 w2258 w2336 w2349 w2380 w2386 w2397 w2402 w2425 w2452 w2466 w2480 w2494 w2504 w2570 w2635 w2700 w2767 w2773 w2778 w2788 w2798 w2808 w2823 w2858 w2882]
          tunnel: [w1875 w2078 w2084 w2103 w2110 w2150 w2181 w2202 w2210 w2215 w2220 w2225 w2247 w2252 w2260 w2338 w2350 w2381 w2387 w2398 w2403 w2437 w2457 w2471 w2485 w2499 w2542 w2607 w2672 w2737 w2768 w2775 w2784 w2794 w2804 w2814 w2828 w2860 w2899] -> w1860
          tunnel: [_ _ _ _ _ _ _ _ _ TRUE _ _ _ _ _ _ _ _ _ _ _ _ _ _ _ _ _ _ _ _ _ _ _ _ _ _ _ _ _] -> w1855
          tunnel: [w1871 w2076 w2083 w2102 w2105 w2147 w2167 w2201 w2208 w2213 w2218 w2223 w2246 w2250 w2259 w2337 w2347 w2379 w2385 w2396 w2401 w2436 w2453 w2467 w2481 w2495 w2539 w2604 w2669 w2734 w2761 w2774 w2782 w2792 w2802 w2812 w2817 w2859 w2892] -> w1859
          tunnel: 250 ("Timeout") -> [w1870 _ _ _ _ _ _ _ _ _ _ _ _ _ _ _ _ _ _ _ _ _ _ _ _ _ _ _ _ _ _ _ _ _ _ _ _ _ _]
          tunnel: w1850 -> [w1869 w2075 w2080 w2092 w2106 w2149 w2176 w2200 w2204 w2211 w2217 w2222 w2243 w2249 w2256 w2333 w2344 w2378 w2383 w2389 w2400 w2435 w2456 w2470 w2484 w2498 w2541 w2606 w2671 w2736 w2762 w2771 w2783 w2793 w2803 w2813 w2827 w2857 w2895]
          tunnel: [w1869 w2075 w2080 w2092 w2106 w2149 w2176 w2200 w2204 w2211 w2217 w2222 w2243 w2249 w2256 w2333 w2344 w2378 w2383 w2389 w2400 w2435 w2456 w2470 w2484 w2498 w2541 w2606 w2671 w2736 w2762 w2771 w2783 w2793 w2803 w2813 w2827 w2857 w2893] -> w1849
          tunnel: w1847 -> [w1868 _ _ _ _ _ _ _ _ _ _ _ _ _ _ _ _ _ _ _ _ _ _ _ _ _ _ _ _ _ _ _ _ _ _ _ _ _ _]
          tunnel: w1845 -> [_ _ _ _ _ _ _ _ _ _ _ _ _ _ _ _ _ _ _ _ _ _ _ _ _ _ _ _ _ _ _ _ _ _ _ _ w2821 _ _]
          tunnel: w1844 -> [_ _ _ _ _ _ _ _ _ _ _ _ _ _ _ _ _ _ _ _ _ _ _ _ _ _ _ _ _ _ _ _ _ _ _ _ w2820 _ _]
          tunnel: w1843 -> [_ _ _ _ _ _ _ _ _ _ _ _ _ _ _ _ _ _ _ _ _ _ _ _ _ _ _ _ _ _ _ _ _ _ _ _ w2819 _ _]
          tunnel: w1842 -> [_ _ _ _ _ _ _ _ _ _ _ _ _ _ _ _ _ _ _ _ _ _ _ _ _ _ _ _ _ _ _ _ _ _ _ _ w2818 _ _]
          tunnel: w1841 -> [_ _ _ _ _ w2145 _ _ _ _ _ _ _ _ _ _ _ _ _ _ _ _ _ _ _ _ _ _ _ _ _ _ _ _ _ _ _ _ _]
          tunnel: w1840 -> [_ _ _ _ _ w2144 _ _ _ _ _ _ _ _ _ _ _ _ _ _ _ _ _ _ _ _ _ _ _ _ _ _ _ _ _ _ _ _ _]
          tunnel: w1839 -> [_ _ _ _ _ w2143 _ _ _ _ _ _ _ _ _ _ _ _ _ _ _ _ _ _ _ _ _ _ _ _ _ _ _ _ _ _ _ _ _]
          tunnel: w1838 -> [_ _ _ _ _ w2142 _ _ _ _ _ _ _ _ _ _ _ _ _ _ _ _ _ _ _ _ _ _ _ _ _ _ _ _ _ _ _ _ _]
          frame "", "Idle" {
            n692 = event shown="[0] Timeout" {
              selector: w1868 -> [_ _ _ _ _ _]
              dyn-events: _ -> [_ _ _ _ _ _]
              timeout: w1870 -> [_ _ _ _ _ _]
              tunnel: w1876 -> [w1884 w1951 w1961 w1975 w2020 w2055]
              tunnel: [w1885 w1950 w1960 w1975 w2020 w2054] -> w1875
              tunnel: w1874 -> [w1880 w1948 w1962 w1977 w2019 w2060]
              tunnel: [w1879 w1949 w1952 w1981 w2014 w2056] -> w1873
              tunnel: w1872 -> [w1882 w1949 w1953 w1981 w2016 w2057]
              tunnel: [w1880 w1948 w1962 w1976 w2018 w2058] -> w1871
              event Timeout {
                n693 = event-data() -> ()  [unwired: 1 in, 1 out]
                n694 = local read "LV Program"() -> (w1878:T25)
                n695 = case shown="Default" w1878 {
                  tunnel: ["Test: Update Display A\nCheck for UI Event" "Test: Update Display A\nTest: Update Display B\nTest: Update Display C\nTest: Update Display D\nCheck for UI Event"] -> w1881
                  frame Default {
                  }
                  frame "PRAT", "HEWH RLT" {
                  }
                }
                n696 = case shown="True" "Start/Pause test" {
                  tunnel: [w1891 w1899] -> w1883
                  tunnel: w1882 -> [w1888 w1903]
                  tunnel: [w1890 w1902] -> w1879
                  tunnel: w1881 -> [w1891 w1901]
                  tunnel: w1880 -> [_ w1898]
                  frame False {
                    n697 = local read "Start Draw Loop"() -> (w1889:bool)
                    n698 = case shown="True" w1889 {
                      tunnel: w1888 -> [w1892 w1894]
                      tunnel: [w1892 w1893] -> w1890
                      frame False {
                      }
                      frame True {
                        n699 = call "UTILITY String Notifier.vi"("Status"=UTILITY_Notifier."Set", "error in (no error)"=w1894, "Set Status"=T8 "Select Test Sequence to Enable Start Button...." ("Message"), "name (unnamed)"="Message") -> ("error out"=w1893:errorcluster)  [unwired: 6 in, 1 out]
                      }
                    }
                  }
                  frame True {
                    n700 = First Call?() -> (First Call?: T/F=w1904:bool)
                    n701 = case shown="True" w1904 {
                      tunnel: w1903 -> [w1911 w1942]
                      tunnel: [w1907 w1941] -> w1902
                      tunnel: w1898 -> [w1910 _]
                      frame False {
                        n702 = while {
                          tunnel: w1910 -> [w1927]
                          shift-right: [w1922] -> w1908
                          shift-left: w1911 -> [w1928]
                          shift-right: [w1918] -> _
                          shift-left: _ -> [w1917]
                          stop <- TRUE stop-if-true
                          n703 = Increment(x=w1917) -> (x+1=w1918:dbl)
                          n704 = Unbundle By Name(w1927) -> ("Station A Display.Display Data (RLT)"=w1926:T32, "Station B Display.Display Data (RLT)"=w1925:T32, "Station C Display.Display Data (RLT)"=w1924:T32, "Station D Display.Display Data (RLT)"=w1923:T32)
                          n705 = local read "Test CompleteD"() -> (w1912:bool)
                          n706 = local read "Test CompleteB"() -> (w1914:bool)
                          n707 = local read "Test CompleteC"() -> (w1913:bool)
                          n708 = local read "Test CompleteA"() -> (w1915:bool)
                          n709 = Quotient & Remainder(x=w1918, y=4) -> (x-y*floor(x/y)=w1919:i32)  [unwired: 1 out]
                          n710 = Equal To 0?(x=w1919) -> (x = 0?=w1916:bool)
                          "Update Heating Message" <- w1916
                          n711 = case shown="True" w1916 {
                            tunnel: w1928 -> [w1929 w1939]
                            tunnel: w1926 -> [_ w1938]
                            tunnel: w1925 -> [_ w1937]
                            tunnel: w1924 -> [_ w1936]
                            tunnel: w1923 -> [_ w1935]
                            tunnel: [w1929 w1934] -> w1922
                            tunnel: w1915 -> [_ w1933]
                            tunnel: w1914 -> [_ w1932]
                            tunnel: w1913 -> [_ w1931]
                            tunnel: w1912 -> [_ w1930]
                            frame False {
                            }
                            frame True {
                              n712 = call "HEWH Update Message.vi"("Display Data (RLT) A"=w1938, "Test CompleteA"=w1933, "Test CompleteB"=w1932, "Test CompleteC"=w1931, "Test CompleteD"=w1930, "Display Data (RLT) B"=w1937, "Display Data (RLT) C"=w1936, "Display Data (RLT) D"=w1935, "error in (no error)"=w1939) -> ("error out"=w1934:errorcluster)  [unwired: 6 in]
                            }
                          }
                        }
                        n713 = call "UTILITY String Notifier.vi"("Status"=UTILITY_Notifier."Set", "error in (no error)"=w1908, "Set Status"="", "name (unnamed)"="Message") -> ("error out"=w1907:errorcluster)  [unwired: 6 in, 1 out]
                      }
                      frame True {
                        w1940 = FALSE ("Show Stand Override Flow Data A")
                        n714 = local write "Show Stand Override Flow Data B"(w1940) -> ()
                        n715 = local write "Show Stand Override Flow Data A"(w1940) -> ()
                        n716 = local write "Show Stand Override Flow Data C"(w1940) -> ()
                        n717 = local write "Show Stand Override Flow Data D"(w1940) -> ()
                        n718 = call "UTILITY String Notifier.vi"("Status"=UTILITY_Notifier."Set", "error in (no error)"=w1942, "Set Status"=T8 "Starting Test...." ("Message"), "name (unnamed)"="Message") -> ("error out"=w1941:errorcluster)  [unwired: 6 in, 1 out]
                      }
                    }
                    n719 = call <vilib>:"Add State(s) to Queue__jki_lib_state_machine.vi"("State(s) in Front (\"\")"="Test: Check Complete", "State(s) in (\"\")"=w1901) -> ("States Out"=w1899:string)  [unwired: 13 in]
                  }
                }
                n720 = call <vilib>:"Add State(s) to Queue__jki_lib_state_machine.vi"("State(s) in Front (\"\")"=w1883, "State(s) in (\"\")"=w1884) -> ("States Out"=w1885:string)  [unwired: 13 in]
              }
              event Panel Close? {
                n721 = event-data() -> ()  [unwired: 1 in, 1 out]
                n722 = call <vilib>:"Add State(s) to Queue__jki_lib_state_machine.vi"("State(s) in Front (\"\")"="Macro: Exit", "State(s) in (\"\")"=w1951) -> ("States Out"=w1950:string)  [unwired: 13 in]
                n723 = event-data("Discard?"=TRUE) -> ()  [unwired: 1 in, 1 out]
              }
              event Menu Selection (User) {
                n724 = event-data() -> ("ItemTag"=w1956:string)  [unwired: 1 in, 6 out]
                n725 = call <vilib>:"Trim Whitespace.vi"("string"=w1956) -> ("trimmed string"=w1958:string)  [unwired: 1 in]
                n726 = call <vilib>:"Trim Whitespace.vi"("string"="Exit") -> ("trimmed string"=w1959:string)  [unwired: 1 in]
                n727 = Equal?(x=w1958, y=w1959) -> (x = y?=w1955:bool)
                n728 = case shown="True" w1955 {
                  tunnel: ["" "Macro: Exit"] -> w1954
                  tunnel: w1953 -> [w1963 w1966]
                  tunnel: [w1963 w1965] -> w1952
                  frame False {
                  }
                  frame True {
                    n729 = for {
                      N: 10 -> [_]
                      shift-right: [w1970] -> w1965
                      shift-left: w1966 -> [w1971]
                      n730 = call "UTILITY Boolean Notifier.vi"("Status"=UTILITY_Notifier."Set", "error in (no error)"=w1971, "Set Status"=TRUE, "name (unnamed)"="Stop Custom Draw") -> ("error out"=w1970:errorcluster)  [unwired: 6 in, 1 out]
                      n731 = Wait Until Next ms Multiple(millisecond multiple=u32 10) -> ()  [unwired: 1 out]
                    }
                  }
                }
                n732 = call <vilib>:"Add State(s) to Queue__jki_lib_state_machine.vi"("State(s) in Front (\"\")"=w1954, "State(s) in (\"\")"=w1961) -> ("States Out"=w1960:string)  [unwired: 13 in]
              }
              event User Event {
                n733 = event-data() -> ()  [unwired: 1 in, 5 out]
                n734 = local read "Station ID to Reset"() -> (w1978:T26)
                n735 = local read "Updated Cycle Count"() -> (w1980:i32)
                n736 = local read "Reset Cycle Count"() -> (w1979:bool)
                n737 = case shown="\"A\", Default" w1978 {
                  tunnel: [w1985 w1993 w2000 w2008] -> w1976
                  tunnel: w1979 -> [w1984 w1992 w2001 w2009]
                  tunnel: w1980 -> [w1983 w1991 w1999 w2007]
                  tunnel: w1977 -> [w1982 w1990 w1998 w2006]
                  frame "A", Default {
                    n738 = case shown="True" w1984 {
                      tunnel: w1982 -> [w1986 w1989]
                      tunnel: [w1986 w1988] -> w1985
                      tunnel: w1983 -> [_ w1987]
                      frame False {
                      }
                      frame True {
                        n739 = Bundle By Name(cluster=w1989, "Station A Display.Display Data (RLT).Cycle Count Display"=w1987) -> (w1988:T97)
                      }
                    }
                  }
                  frame "B" {
                    n740 = case shown="True" w1992 {
                      tunnel: w1990 -> [w1994 w1997]
                      tunnel: [w1994 w1996] -> w1993
                      tunnel: w1991 -> [_ w1995]
                      frame False {
                      }
                      frame True {
                        n741 = Bundle By Name(cluster=w1997, "Station B Display.Display Data (RLT).Cycle Count Display"=w1995) -> (w1996:T97)
                      }
                    }
                  }
                  frame "C" {
                    n742 = case shown="True" w2001 {
                      tunnel: w1998 -> [w2002 w2005]
                      tunnel: [w2002 w2004] -> w2000
